vi "SV TDMS Write Speed Profile (1 Ch).vi"(0 "tdms file":refnum<k34>, 5 "group name in":string="SpeedProfile", 7 "channel name in":string="Channel0", 9 "speed profile":T2 {"speed [RPM]" format="%.2f"; "time [s]" format="%.2f"}, 11 "error in":errorcluster, 13 "speed position info":T1) -> (4 "tdms file out":refnum<k34>, 6 "group name out":string, 8 "channel name out":string, 15 "error out":errorcluster)   [LabVIEW 2017]
doc: "Writes data to the specified .tdms file in a format specific to the polymorphic instance. Wire data to the <B>scaled signal [EU]</B> input to determine the polymorphic instance to use or manually select the instance."
uses:
  <vilib>/addons/_NISVFA/_Shared subVIs/Controls/svc_Speed Profile.ctl
  <vilib>/addons/_NISVFA/_Shared subVIs/Controls/svc_Position Info.ctl
  <vilib>/addons/_NISVFA/_Shared subVIs/Controls/NI Function Type.ctl
  <vilib>/addons/_NISVFA/_Shared subVIs/Controls/NI Function SubType.ctl
  <vilib>/addons/_NISVFA/_Shared subVIs/Controls/svc_X-Axis Units.ctl
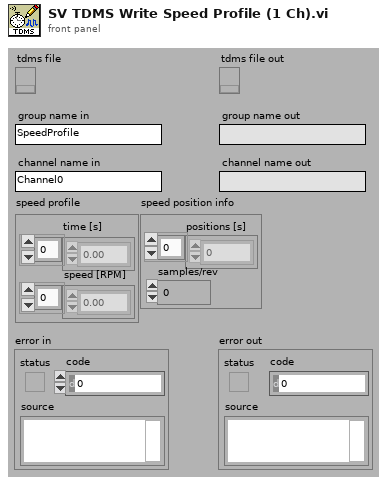
[diagram p1: front panel]
types:
  T1 = typedef "svc_Position Info.ctl" = cluster{"positions [s]":dbl[], "samples/rev":dbl}
  T2 = typedef "svc_Speed Profile.ctl" = cluster{"time [s]":dbl[], "speed [RPM]":dbl[]}
  T3 = typedef "NI Function Type.ctl" = u16
  T4 = typedef "NI Function SubType.ctl" = u16
  T5 = typedef "svc_X-Axis Units.ctl" = u16
  T6 = cluster{"function type":T3, "function subtype":T4, "X-domain":T5}
  T7 = cluster{"X-axis label":string, "X-unit string":string, "Y-axis label":string, "Y-unit string":string}
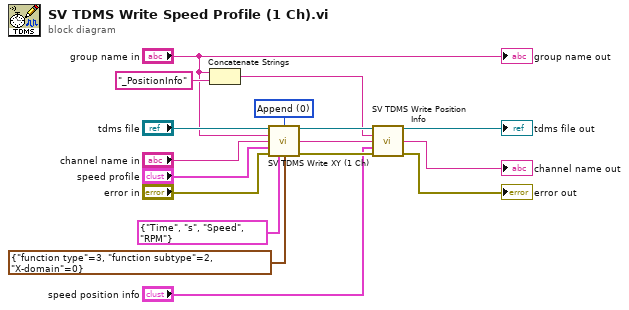
[diagram p0: block diagram]
diagram:
  w12 = u16 0 items=["Append", "New group", "Overwrite"] ("write mode")
  n1 = Concatenate Strings("group name in", "_PositionInfo" ("string")) -> (w4:string)
  n2 = call <vilib>:"SV TDMS Write XY (1 Ch).vi"("tdms file"="tdms file", "write mode"=w12, "group name in"="group name in", "channel name in"="channel name in", "XY"="speed profile", "error in"="error in", "unit info"=T7 {"X-axis label"="Time", "X-unit string"="s", "Y-axis label"="Speed", "Y-unit string"="RPM"} ("XY info"), "function info"=T6 {"function type"=3, "function subtype"=2, "X-domain"=0}) -> ("tdms file out"=w10:refnum<k34>, "channel name out"=w3:string, "error out"=w8:errorcluster)  [unwired: 4 in, 1 out]
  n3 = call <vilib>:"SV TDMS Write Position Info.vi"("tdms file"=w10, "group name in"=w4, "channel name in"=w3, "speed position info"="speed position info", "error in (no error)"=w8) -> ("tdms file out"=→"tdms file out":refnum<k34>, "channel name out"=→"channel name out":string, "error out"=→"error out":errorcluster)  [unwired: 7 in, 1 out]
  "group name out" <- "group name in"
